vi "init.vi"(8 "error in (no error)":errorcluster, 11 "Hardware in":refnum<class "Hardware.lvclass">) -> (0 "error out":errorcluster, 3 "Hardware out":refnum<class "Hardware.lvclass">)   [LabVIEW 2026, in "Hardware.lvlib" / "Hardware.lvclass"]
uses:
  Hardware.lvclass
  Hardware.lvclass/Hardware.ctl
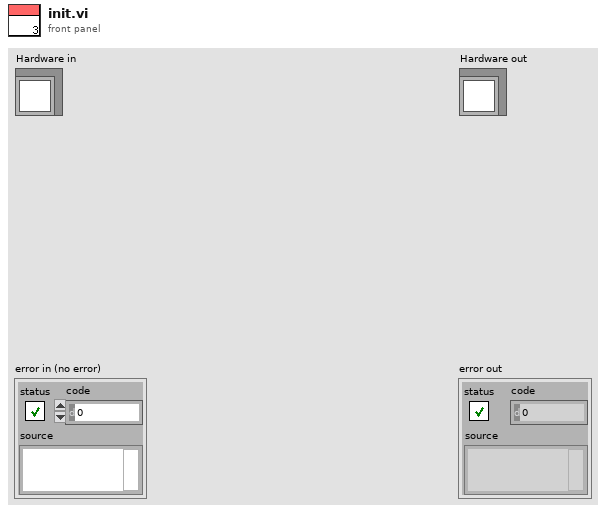
[diagram p1: front panel]
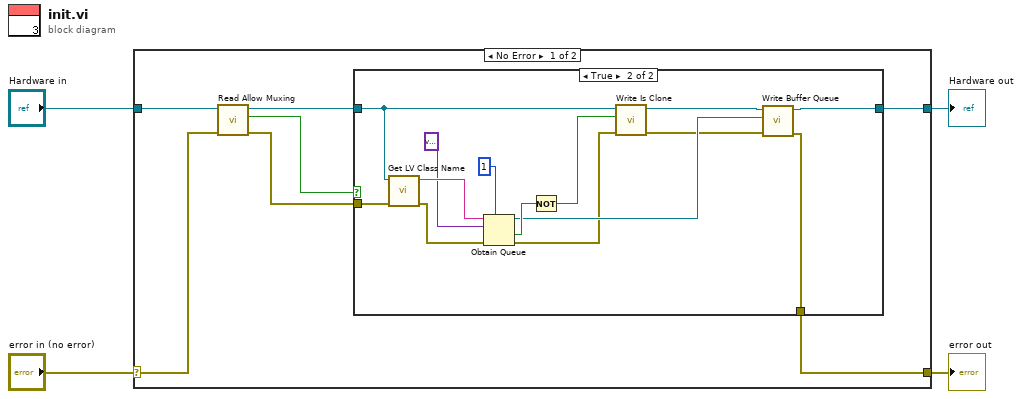
[diagram p0: block diagram]
diagram:
  n1 = case shown="No Error" "error in (no error)" {
    selector: "error in (no error)" -> [w6 w29]
    tunnel: [w10 w29] -> w3
    tunnel: [w11 w28] -> w1
    tunnel: "Hardware in" -> [w9 w28]
    frame No Error {
      n2 = call "Read Allow Muxing.vi"("error in (no error)"=w6, "Hardware in"=w9) -> ("error out"=w5:errorcluster, "Allow Muxing"=w7:bool, "Hardware out"=w8:refnum<class "Hardware.lvclass">)  [unwired: 7 in]
      n3 = case shown="True" w7 {
        tunnel: [w13 w20] -> w11
        tunnel: [w12 w17] -> w10
        tunnel: w8 -> [w13 w16]
        tunnel: w5 -> [w12 w15]
        frame False {
        }
        frame True {
          n4 = call <vilib>:"Get LV Class Name.vi"("error in (no error)"=w15, "object"=w16) -> ("error out"=w14:errorcluster, "class name"=w26:string)  [unwired: 8 in]
          n5 = Obtain Queue(max queue size (-1, unlimited)=1, name (unnamed)=w26, element data type=variant, error in (no error)=w14) -> (queue out=w23:refnum<queue>, created new?=w25:bool, error out=w19:errorcluster)  [unwired: 1 in]
          n6 = Not(x=w25) -> (.not. x?=w24:bool)
          n7 = call "Write Is Clone.vi"("error in (no error)"=w19, "Is Clone?"=w24, "Hardware in"=w16) -> ("error out"=w18:errorcluster, "Hardware out"=w21:refnum<class "Hardware.lvclass">)  [unwired: 7 in]
          n8 = call "Write Buffer Queue.vi"("error in (no error)"=w18, "Buffer Queue"=w23, "Hardware in"=w21) -> ("error out"=w17:errorcluster, "Hardware out"=w20:refnum<class "Hardware.lvclass">)  [unwired: 7 in]
        }
      }
    }
    frame Error {
    }
  }
  "error out" <- w3
  "Hardware out" <- w1
